vi "Fpga-ItchParser-TestHarness.vi"   [LabVIEW 2016]
uses:
  <vilib>/Platform/TimedLoop/XDataNode/timing_clust.ctl
  <vilib>/Platform/TimedLoop/XDataNode/nitl_modes.ctl
  <vilib>/Platform/TimedLoop/XDataNode/wakeup.ctl
  <vilib>/rvi/Emulation/niFpgaSctlEmulationGetInTimedLoop.vi
  <vilib>/rvi/Emulation/niFpgaEmulationReportErrorSimple.vi
  <vilib>/rvi/Emulation/niFpgaGetClockAttributes.vi
  <vilib>/rvi/Emulation/niFpgaCriticalErrorInLSC.vi
  <vilib>/rvi/interface/RandomDataEmulation/niFpgaRandomDataHandleErrors.vi
  <vilib>/rvi/Emulation/niFpgaEmulationIsFPGAContextNoSignature.vi
  <vilib>/rvi/errors/niFpgaSetErrorForExecOnDevCompSimple.vi
  <vilib>/rvi/eio/common/nirviEmuReportErrorAndStop.vi
  <vilib>/rvi/DataTransferAndStorage/Container/Common/niFpgaContainerGetUniqueNameForEmu.vi
  <vilib>/rvi/FIFO/Fifo_Resource/nirvififoEmulationSetSize.vi
  <vilib>/rvi/FIFO/Fifo_Resource/nirviFifoEmulationQueueMgr.vi
  <instcachedir>/0/nirviFifoEmulationQueueMgr_E5CAEC123FF24DC58D834DCA3CDAA9B5.lvgen/nirviFifoEmulationQueueMgr_E5CAEC123FF24DC58D834DCA3CDAA9B5_008.vi
  <vilib>/rvi/FIFO/Fifo_Resource/nirvififoEmulationDetermineInputValidOut.vi
  <vilib>/rvi/FIFO/Fifo_Resource/nirvififoEmulationCreateLock.vi
  <vilib>/rvi/Emulation/niFpgaProcessEmulError.vi
  <vilib>/rvi/FIFO/Fifo_Resource/nirvififoEmulationObtainLock.vi
  <vilib>/rvi/FIFO/Fifo_Resource/nirvififoEmulationReleaseLock.vi
  <vilib>/rvi/occurrence/nirviWaitOnOccurrenceBase.vi
  <vilib>/rvi/errors/nirviReportUnexpectedCaseInternalError.vi
  <vilib>/rvi/errors/nirviReportUnexpectedCaseInternalError (U32).vi
  <instcachedir>/0/nirviFifoEmulationQueueMgr_E5CAEC123FF24DC58D834DCA3CDAA9B5.lvgen/nirviFifoEmulationQueueMgr_E5CAEC123FF24DC58D834DCA3CDAA9B5_009.vi
  <vilib>/Utility/error.llb/Clear Errors.vi
  <vilib>/Platform/TimedLoop/XDataNode/XDataNode.xnode
  <vilib>/rvi/DataTransferAndStorage/Container/XNode/niFpgaContainer.xnode
  <vilib>/rvi/interface/RandomDataEmulation/nirviRandomDataFpgaReadWriteTemplate.vi
  <vilib>/rvi/FIFO/Fifo_Resource/nirvififoEmulationWrite.vi
  <vilib>/rvi/FIFO/Fifo_Resource/nirvififoEmulationRead.vi
  <vilib>/Platform/TimedLoop/XDataNode/XDNodeRunTimeDep.lvlib
types:
  T1 = cluster{"Operation":enum16{"Noop", "GetAll", "AddOrder", "DeleteOrder"}, "Cluster":cluster{"Side":u16, "OrderRefNum":u64, "Price":u32, "Shares":u32}}
  T2 = typedef "XDNodeRunTimeDep.lvlib/timing_clust.ctl" = cluster{"Expected End [f-1]":u64, "Actual End [f-1]":u64, "Finished Late? [f-1]":bool, "Expected End [i-1]":u64, "Actual End [i-1]":u64, "Finished Late? [i-1]":bool, "Expected Start [i]":u64, "Actual Start [i]":u64, "Expected Start [f]":u64, "Actual Start [f]":u64, "Source Name":string, "Structure Name":string, "Period":i64, "Deadline":i64, "Offset":i64, "Start":i64, "Priority":i32, "Timeout":i32, "Mode":T3, "Wakeup Reason":T4, "Error":errorcluster, "Source Type":string, "Secondary Source Type":string, "Global End Time":u64, "Global Start Time":u64, "Frame Duration":u64, "Iteration Duration":u64, "Assigned CPU":i32, "I/O Scan Engine Mode":u32}
  T3 = typedef "XDNodeRunTimeDep.lvlib/nitl_modes.ctl" = enum32{"No Change", "Process missed periods, maintain original phase", "Discard missed periods, maintain original phase", "Process missed periods, ignore original phase", "Discard missed periods, ignore original phase"}
  T4 = typedef "XDNodeRunTimeDep.lvlib/wakeup.ctl" = enum32{"Normal", "Aborted", "Asynchronous wakeup", "Timing source error", "Timed loop error", "Timeout"}
  T5 = enum16{"Noop", "GetAll", "AddOrder", "DeleteOrder"}
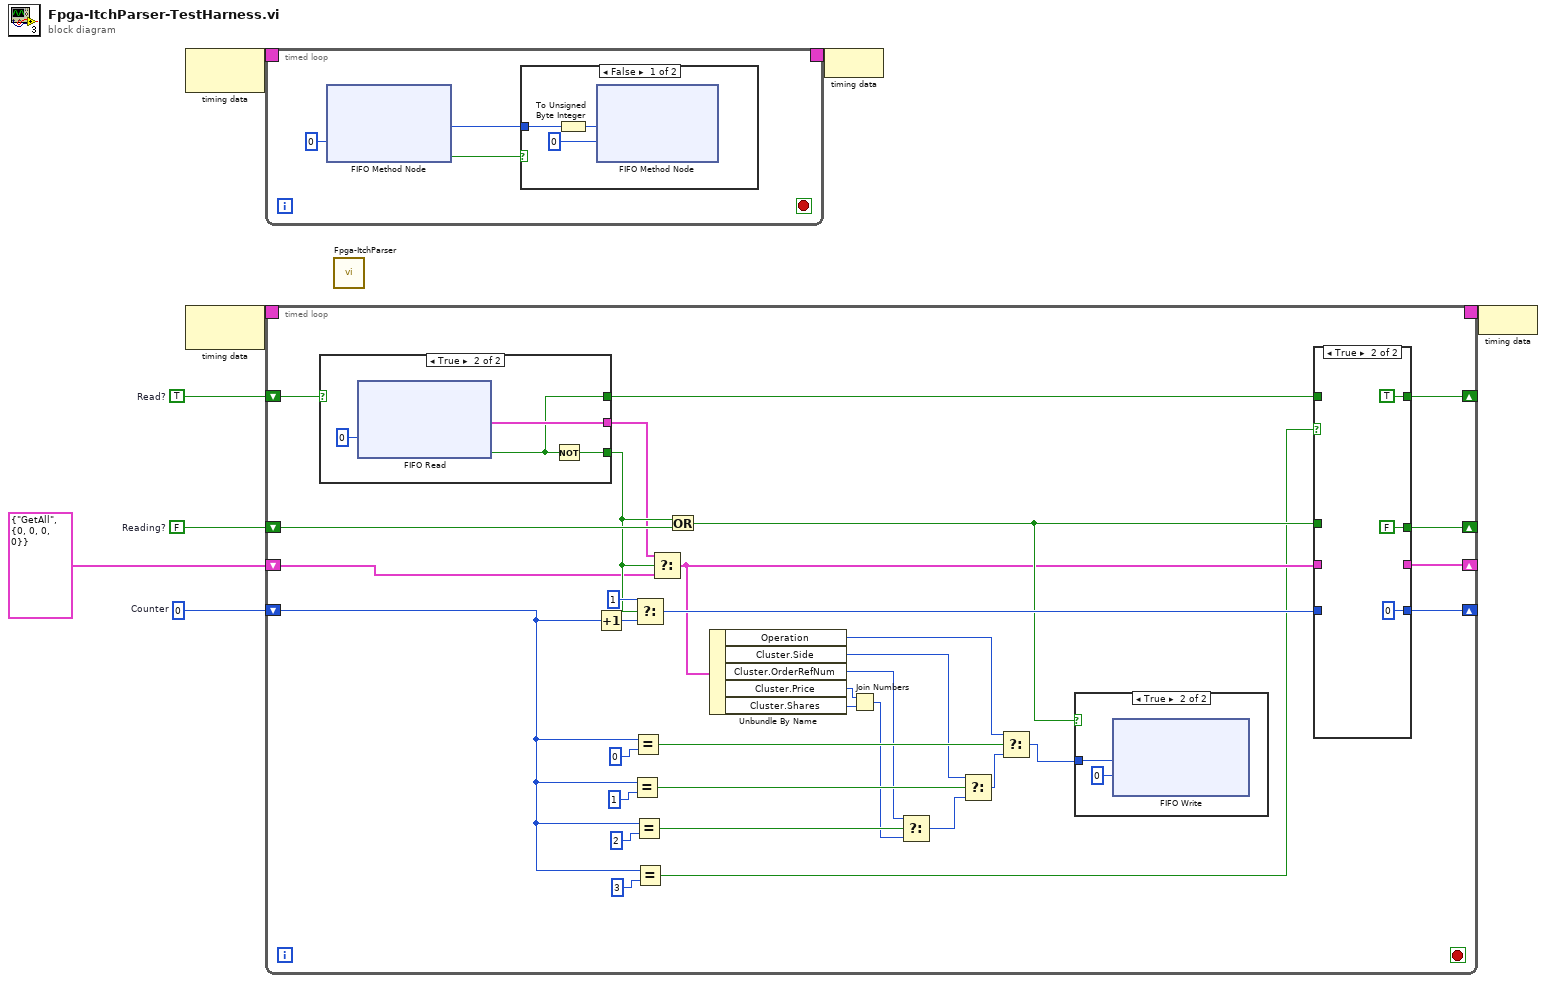
[diagram p0: block diagram]
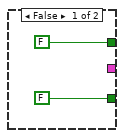
[diagram p4: hidden frame]
diagram:
  w2 = FALSE  # Reading?
  w3 = i16 0  # Counter
  w4 = TRUE  # Read?
  n1 = node-c288() -> (w8:T2)  [unwired: 1 in]
  n2 = node-c288() -> (w6:T2)  [unwired: 1 in]
  n3 = timed-loop {
    timing: w8 -> [_]
    timing-out: [_] -> w7
    stop <- _ stop-if-true
    n4 = xnode ("FIFO Method Node")("Timeout"=0) -> ("Element"=w9:u8, "Timed Out?"=w10:bool)  [unwired: 1 in, 1 out]
    n5 = case shown="False" w10 {
      tunnel: w9 -> [w13 _]
      frame False {
        n6 = To Unsigned Byte Integer(number=w13) -> (unsigned 8bit integer=w12:u8)
        n7 = xnode ("FIFO Method Node")("Element"=w12, "Timeout"=0) -> ()  [unwired: 1 in, 2 out]
      }
      frame True {
      }
    }
  }
  n8 = timed-loop {
    timing: w6 -> [_]
    timing-out: [_] -> w5
    shift-right: [w47] -> _
    shift-left: w4 -> [w48]
    shift-right: [w45] -> _
    shift-left: w3 -> [w24]
    shift-right: [w43] -> _
    shift-left: w2 -> [w44]
    shift-right: [w37] -> _
    shift-left: T1 {"Operation"=enum."GetAll", "Cluster"={"Side"=0, "OrderRefNum"=0, "Price"=0, "Shares"=0}} ("OrderBookCommand") -> [w36]
    stop <- _ stop-if-true
    n9 = case shown="True" w48 {
      tunnel: [_ w63] -> w39
      tunnel: [FALSE ("Timed Out?") w62] -> w40
      tunnel: [FALSE w61] -> w46
      frame False {
      }
      frame True {
        n10 = xnode "FIFO Read"("Timeout"=0) -> ("Element"=w63:T1, "Timed Out?"=w61:bool)  [unwired: 1 in, 1 out]
        n11 = Not(x=w61) -> (.not. x?=w62:bool)
      }
    }
    n12 = Increment(x=w24) -> (x+1=w49:i16)
    n13 = Equal?(x=w24, y=i16 1) -> (x = y?=w30:bool)
    n14 = Equal?(x=w24, y=i16 0) -> (x = y?=w32:bool)
    n15 = Equal?(x=w24, y=i16 2) -> (x = y?=w21:bool)
    n16 = Select(t=i16 1, s=w40, f=w49) -> (s? t:f=w41:i16)
    n17 = Equal?(x=w24, y=i16 3) -> (x = y?=w22:bool)
    n18 = Select(t=w39, s=w40, f=w36) -> (s? t:f=w28:T1)
    n19 = Or(x=w40, y=w44) -> (x .or. y?=w38:bool)
    n20 = Unbundle By Name(w28) -> ("Operation"=w27:T5, "Cluster.Side"=w26:u16, "Cluster.OrderRefNum"=w20:u64, "Cluster.Price"=w19:u32, "Cluster.Shares"=w18:u32)
    n21 = Join Numbers(hi=w19, lo=w18) -> ((hi.lo)=w17:u64)
    n22 = Select(t=w20, s=w21, f=w17) -> (s? t:f=w23:u64)
    n23 = Select(t=w26, s=w30, f=w23) -> (s? t:f=w31:u64)
    n24 = Select(t=w27, s=w32, f=w31) -> (s? t:f=w29:u64)
    n25 = case shown="True" w38 {
      tunnel: w29 -> [_ w50]
      frame False {
      }
      frame True {
        n26 = xnode "FIFO Write"("Element"=w50, "Timeout"=0) -> ()  [unwired: 1 in, 2 out]
      }
    }
    n27 = case shown="True" w22 {
      tunnel: [w55 TRUE ("Timed Out?")] -> w47
      tunnel: w46 -> [w55 _]
      tunnel: w41 -> [w54 _]
      tunnel: [w54 i16 0 ("Counter")] -> w45
      tunnel: w38 -> [w53 _]
      tunnel: [w53 FALSE] -> w43
      tunnel: [w52 _] -> w37
      tunnel: w28 -> [w52 _]
      frame False {
      }
      frame True {
      }
    }
  }
  n28 = call "Fpga-ItchParser.vi"() -> ()  [unwired: 12 in]
  n29 = node-c288(w7) -> ()
  n30 = node-c288(w5) -> ()
